vi "DAQNavi Create Channel(CO-Frequency).vi"(0 "task in":i32=-1, 5 "physical channels":string="DemoDevice,BID#0/cntr0", 7 "frequency":dbl=-1.0, 11 "error in (no error)":errorcluster) -> (4 "task out":i32, 15 "error out":errorcluster)   [LabVIEW 2020]
uses:
  DAQNavi_LV.dll
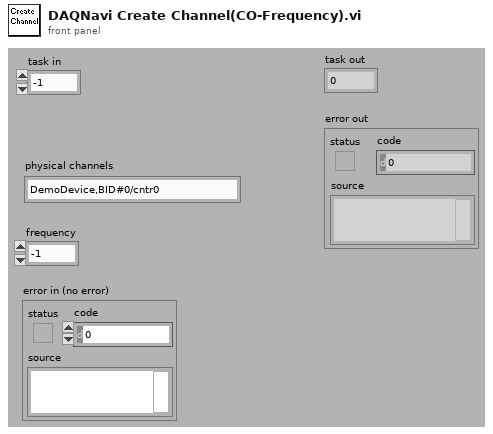
[diagram p1: front panel]
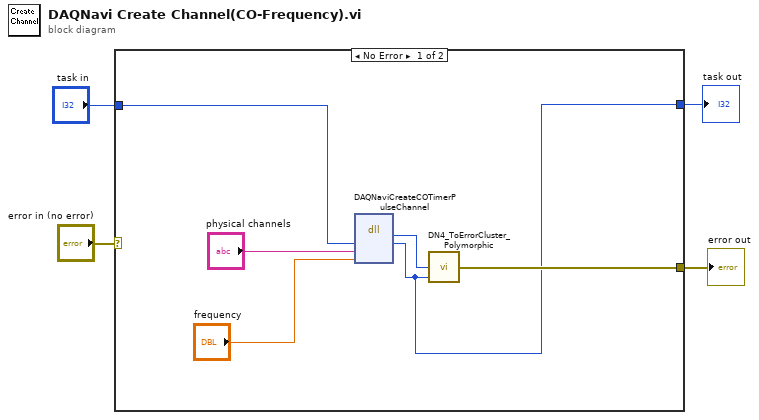
[diagram p0: block diagram]
diagram:
  n1 = case shown="No Error" "error in (no error)" {
    selector: "error in (no error)" -> [_ w11]
    tunnel: "task in" -> [w10 w12]
    tunnel: [w5 w12] -> w2
    tunnel: [w6 w11] -> w1
    frame No Error {
      n2 = dll-call lib="DAQNavi_LV.dll" fn="DAQNaviCreateCOTimerPulseChannel"("taskID"=w10, "physicalChannel"="physical channels", "frequency"="frequency") -> ("return type"=w8:i32, "taskID"=w5:i32)  [unwired: 5 in, 2 out]
      n3 = call "DN4_ToErrorCluster_Polymorphic.vi"("task id"=w5, "error code"=w8) -> ("error out"=w6:errorcluster)  [unwired: 3 out]
    }
    frame Error {
    }
  }
  "error out" <- w1
  "task out" <- w2
